vi "ChkOnTarget.vi"(1 "Prec":dbl, 2 "TargetPos":dbl, 3 "CurrPos":dbl) -> (0 "In Range?":bool)   [LabVIEW 2015]
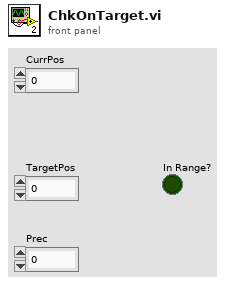
[diagram p1: front panel]
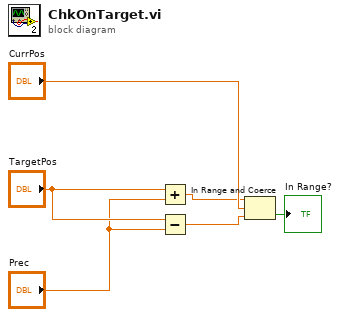
[diagram p0: block diagram]
diagram:
  n1 = Add(x="TargetPos", y="Prec") -> (x+y=w3:dbl)
  n2 = Subtract(x="TargetPos", y="Prec") -> (x-y=w2:dbl)
  n3 = In Range and Coerce(upper limit=w3, x="CurrPos", lower limit=w2) -> (In Range?=→"In Range?":bool)  [unwired: 1 out]
